vi "String to TOD Byte Stream.vi"(8 "error in (no error)":errorcluster, 10 "Value":string) -> (0 "error out":errorcluster, 2 "Byte Stream":u8[](array[numeric]))   [LabVIEW 2018, in "TwinCAT ADS.lvclass"]
uses:
  TwinCAT ADS.lvclass
  TwinCAT.Ads
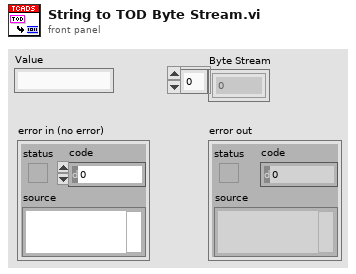
[diagram p1: front panel]
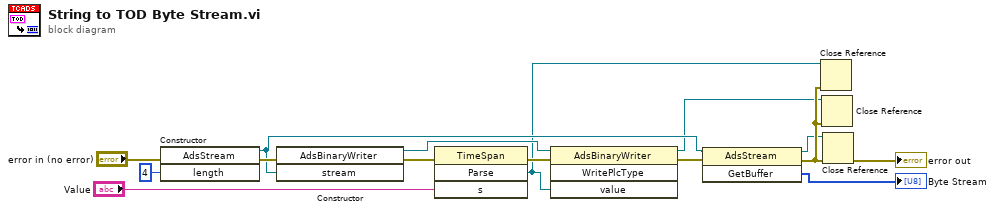
[diagram p0: block diagram]
diagram:
  n1 = constructor class="AdsStream"(error in="error in (no error)", "length"=4) -> (reference out=w8:refnum<k24>, error out=w15:errorcluster)  [unwired: 2 in, 2 out]
  n2 = constructor class="AdsBinaryWriter"(error in=w15, "stream"=w8) -> (reference out=w10:refnum<k24>, error out=w12:errorcluster)  [unwired: 2 in, 2 out]
  n3 = invoke class="TimeSpan" method="Parse"(error in=w12, "s"="Value") -> (error out=w13:errorcluster, "Parse"=w2:refnum<k24>)  [unwired: 2 in, 2 out]
  n4 = invoke class="AdsBinaryWriter" method="WritePlcType"(reference=w10, error in=w13, "value"=w2) -> (reference out=w3:refnum<k24>, error out=w9:errorcluster)  [unwired: 1 in, 2 out]
  n5 = invoke class="AdsStream" method="GetBuffer"(reference=w8, error in=w9) -> (reference out=w4:refnum<k24>, error out=w5:errorcluster, "GetBuffer"=→"Byte Stream":u8[])  [unwired: 1 in]
  n6 = Close Reference(reference=w2, error in (no error)=w5) -> ()  [unwired: 1 out]
  n7 = Close Reference(reference=w3, error in (no error)=w5) -> ()  [unwired: 1 out]
  n8 = Close Reference(reference=w4, error in (no error)=w5) -> (error out=→"error out":errorcluster)
